vi "Spline_fit.vi"(0 "Input Y array":dbl[](array[numeric]) format="%.4f", 2 "Input X array":dbl[](array[numeric]) format="%.3f", 5 "Point selector":cluster{"Y":dbl, "X":dbl, "switch":bool}[](array[cluster]) {"X" format="%.2f"; "Y" format="%.2f"}) -> (4 "Curve fit":dbl[][](array[numeric]) format="%.2f", 6 "Calib const":string[][](array[string]), 7 "Calibration plot":cluster{cluster{dbl, dbl}[]}[](graph), 8 "Point selector":cluster{"Y":dbl, "X":dbl, "switch":bool}[](array[cluster]) {"X" format="%.2f"; "Y" format="%.2f"})   [LabVIEW 2010]
uses:
  <vilib>/Analysis/NI_AALPro.lvlib
panel:
  in  "Type":cluster{"Y":dbl, "X":dbl, "switch":bool}={"Y"=10.144154930121, "X"=9.20412, "switch"=FALSE} {"X" format="%.2f"; "Y" format="%.2f"}
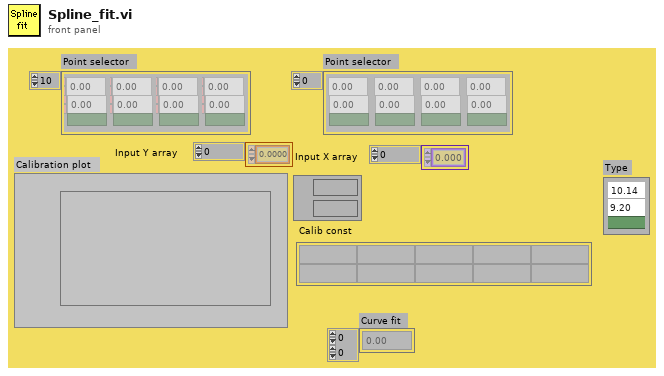
[diagram p1: front panel]
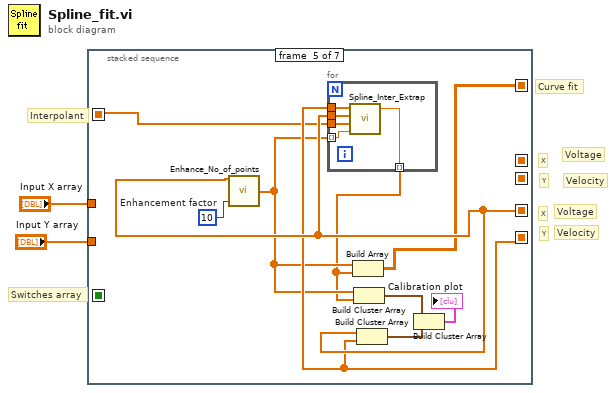
[diagram p0: block diagram]
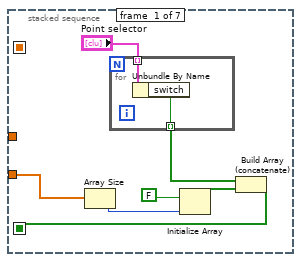
[diagram p2: hidden frame]
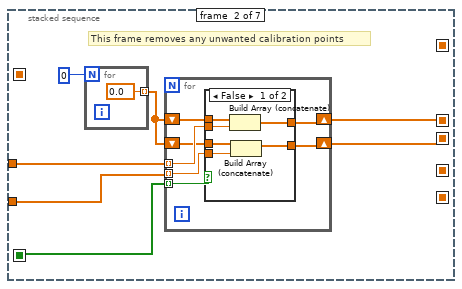
[diagram p3: hidden frame]
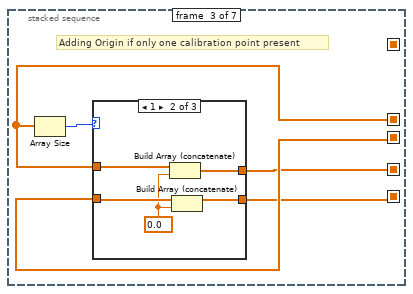
[diagram p5: hidden frame]
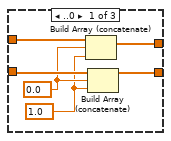
[diagram p6: hidden frame]
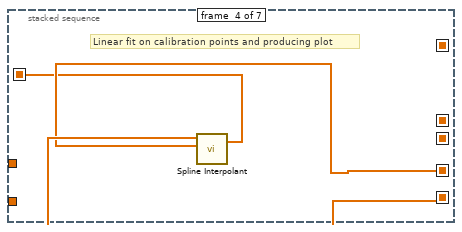
[diagram p8: hidden frame]
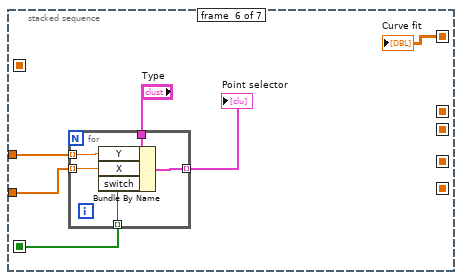
[diagram p9: hidden frame]
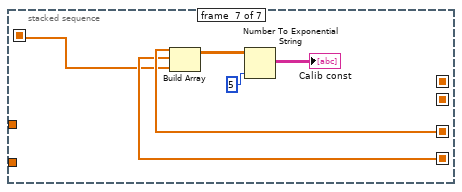
[diagram p10: hidden frame]
diagram:
  # "Curve fit"
  # "Y"
  # "X"
  # "Interpolant"
  # "Voltage"
  # "Velocity"
  # "Velocity"
  # "Voltage"
  # "Switches array"
  # "X"
  # "Y"
  n1 = stacked-sequence {
    seq-local: [_ w16 _ _ _ _ _] -> [_ _ w36 _ _ _ _]
    seq-local: [_ w15 _ _ _ _ _] -> [_ _ w39 _ _ _ _]
    seq-local: [_ _ w37 _ _ _ _] -> [_ _ _ w55 w60 _ w86]
    seq-local: [_ _ w38 _ _ _ _] -> [_ _ _ w54 w61 _ w87]
    seq-local: [w7 _ _ _ _ _ _] -> [_ w12 _ _ _ w73 _]
    seq-local: [_ _ _ w53 _ _ _] -> [_ _ _ _ w59 _ w85]
    seq-local: [_ _ _ _ w56 _ _] -> [_ _ _ _ _ w71 _]
    tunnel: "Input Y array" -> [w3 w13 _ _ _ w74 _]
    tunnel: "Input X array" -> [_ w14 _ _ _ w75 _]
    frame #0 {
      n2 = Array Size(array=w3) -> (size(s)=w5:i32)
      n3 = for {
        tunnel: "Point selector" -> [w11] mode=indexing
        tunnel: [w10] -> w8 mode=indexing
        n4 = Unbundle By Name(w11) -> ("switch"=w10:bool)
      }
      n5 = Initialize Array(FALSE, w5) -> (w4:bool[])
      n6 = Build Array (concatenate)(w8, w4) -> (w7:bool[])
    }
    frame #1 {
      # "This frame removes any unwanted calibration points"
      n7 = for {
        N: 0 -> [_]
        tunnel: [0.0] -> w17 mode=indexing
      }
      n8 = for {
        shift-right: [w20] -> w15
        shift-left: w17 -> [w22]
        shift-right: [w21] -> w16
        shift-left: w17 -> [w23]
        tunnel: w12 -> [w24] mode=indexing
        tunnel: w13 -> [w25] mode=indexing
        tunnel: w14 -> [w26] mode=indexing
        n9 = case shown="False" w24 {
          tunnel: [w27 w33] -> w20
          tunnel: [w28 w34] -> w21
          tunnel: w22 -> [w29 w33]
          tunnel: w23 -> [w30 w34]
          tunnel: w25 -> [w31 _]
          tunnel: w26 -> [w32 _]
          frame False {
            n10 = Build Array (concatenate)(w30, w32) -> (w28:dbl[])
            n11 = Build Array (concatenate)(w29, w31) -> (w27:dbl[])
          }
          frame True {
          }
        }
      }
    }
    frame #2 {
      # "Adding Origin if only one calibration point present"
      n12 = Array Size(array=w36) -> (size(s)=w35:i32)
      n13 = case shown="1" w35 {
        tunnel: [w41 w46 w51] -> w37
        tunnel: [w42 w47 w52] -> w38
        tunnel: w39 -> [w44 w49 w51]
        tunnel: w36 -> [w45 w50 w52]
        frame ..0 {
          w40 = 1.0
          w43 = 0.0
          n14 = Build Array (concatenate)(w45, w43, w40) -> (w42:dbl[])
          n15 = Build Array (concatenate)(w44, w43, w40) -> (w41:dbl[])
        }
        frame 1 {
          w48 = 0.0
          n16 = Build Array (concatenate)(w50, w48) -> (w47:dbl[])
          n17 = Build Array (concatenate)(w49, w48) -> (w46:dbl[])
        }
        frame 2.. {
        }
      }
    }
    frame #3 {
      # "Linear fit on calibration points and producing plot"
      n18 = call <vilib>:"Spline Interpolant.vi"("X"=w54, "Y"=w55) -> ("Interpolant"=w53:dbl[])  [unwired: 2 in, 1 out]
    }
    frame #4 {
      w62 = 10  # Enhancement factor
      n19 = call "Enhance_No_of_points.vi"("Enhancement factor"=w62, "Input"=w61) -> ("Output"=w58:dbl[])  [unwired: 3 in]
      n20 = for {
        tunnel: w61 -> [w70]
        tunnel: w60 -> [w69]
        tunnel: w59 -> [w68]
        tunnel: w58 -> [w67] mode=indexing
        tunnel: [w66] -> w57 mode=indexing
        n21 = call "Spline_Inter_Extrap.vi"("Y calib points"=w69, "X calib points"=w70, "Calib constants"=w68, "Ch voltage"=w67) -> ("Output value"=w66:dbl)  [unwired: 2 in, 1 out]
      }
      n22 = Build Array(w58, w57) -> (w56:dbl[][])
      n23 = Build Cluster Array(w58, w57) -> (w65:cluster{dbl, "Output value":dbl}[])
      n24 = Build Cluster Array(w61, w60) -> (w64:cluster{dbl, dbl}[])
      n25 = Build Cluster Array(w65, w64) -> (→"Calibration plot":cluster{cluster{dbl, "Output value":dbl}[]}[])
    }
    frame #5 {
      n26 = for {
        tunnel: "Type" -> [w81]
        tunnel: w75 -> [w80] mode=indexing
        tunnel: w74 -> [w79] mode=indexing
        tunnel: w73 -> [w78] mode=indexing
        tunnel: [w77] -> w72 mode=indexing
        n27 = Bundle By Name(cluster=w81, "Y"=w80, "X"=w79, "switch"=w78) -> (w77:cluster{"Y":dbl, "X":dbl, "switch":bool})
      }
      "Point selector" <- w72
      "Curve fit" <- w71
    }
    frame #6 {
      n28 = Build Array(w87, w86, w85) -> (w83:dbl[][])
      n29 = Number To Exponential String(number=w83, precision (6)=i16 5) -> (E-format string=→"Calib const":string[][])  [unwired: 2 in]
    }
  }
